vi "PassWrapper.vi"(11 "cPass":bool) -> (2 "Perform?":bool, 3 "Subsystem:\nGround (T)\nElevated (F)":bool)   [LabVIEW 2013]
doc: "Determines which pass method to use and whether to actually call the pass VI.\n\nAccepts the raw controller input (<B>cPass</B>).\nA <B>single</B> button press will select the <B>Ground Pass</B> (True).\nA <B>double</B> button press (i.e. double click) will select the <B>Elevated Pass</B> (False).\nAfter a small delay (250 ms), the VI will output True from <B>Perform?</B>, indicating input can be passed to the Toggle / Pass vi (in a nested case structure)."
uses:
  PassState.ctl
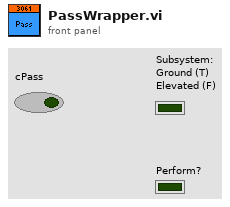
[diagram p1: front panel]
types:
  T1 = typedef "PassState.ctl" = enum16{"Idle", "SingleClick", "DoubleClick", "SelectPass", "Do"}
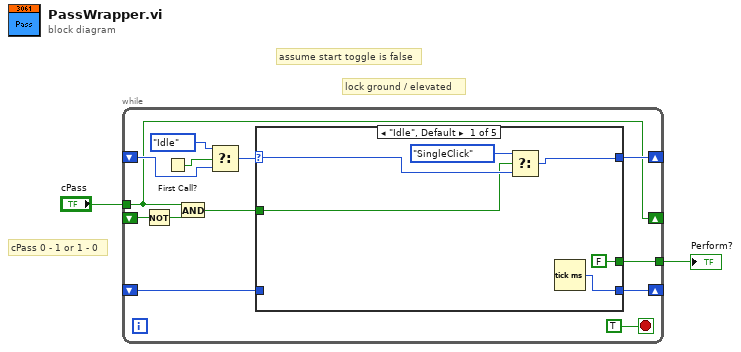
[diagram p0: block diagram]
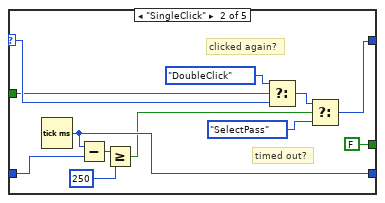
[diagram p2: hidden frame]
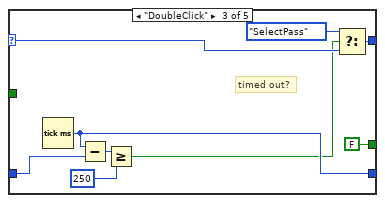
[diagram p3: hidden frame]
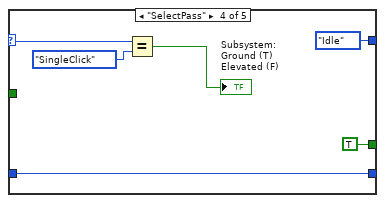
[diagram p4: hidden frame]
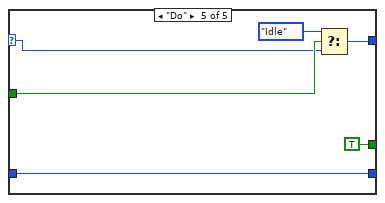
[diagram p5: hidden frame]
diagram:
  # "cPass 0 - 1 or 1 - 0"
  # "assume start toggle is false"
  # "lock ground / elevated"
  n1 = while {
    shift-right: [w10] -> _
    shift-left: _ -> [w11]
    shift-right: [w9] -> _
    shift-left: _ -> [w8]
    tunnel: [w7] -> w2
    shift-right: [w3] -> _
    shift-left: _ -> [w5]
    tunnel: "cPass" -> [w3]
    stop <- TRUE stop-if-true
    n2 = Not(x=w5) -> (.not. x?=w6:bool)
    n3 = First Call?() -> (First Call?: T/F=w14:bool)
    n4 = And(x=w3, y=w6) -> (x .and. y?=w4:bool)
    n5 = Select(t=PassState."Idle", s=w14, f=w11) -> (s? t:f=w12:T1)
    n6 = case shown="\"Idle\", Default" w12 {
      selector: w12 -> [w21 w23 w37 w46 w51]
      tunnel: [w20 w32 w38 PassState."Idle" w49] -> w10
      tunnel: [w18 w27 w39 w48 w53] -> w9
      tunnel: w8 -> [_ w28 w40 w48 w53]
      tunnel: [FALSE FALSE FALSE TRUE TRUE] -> w7
      tunnel: w4 -> [w16 w22 _ _ w52]
      frame "Idle", Default {
        n7 = Select(t=PassState."SingleClick", s=w16, f=w21) -> (s? t:f=w20:T1)
        n8 = Tick Count (ms)() -> (millisecond timer value=w18:u32)
      }
      frame "SingleClick" {
        # "timed out?"
        # "clicked again?"
        n9 = Tick Count (ms)() -> (millisecond timer value=w27:u32)
        n10 = Subtract(x=w27, y=w28) -> (x-y=w30:u32)
        n11 = Greater Or Equal?(x=w30, y=u32 250) -> (x >= y?=w26:bool)
        n12 = Select(t=PassState."DoubleClick", s=w22, f=w23) -> (s? t:f=w33:T1)
        n13 = Select(t=w33, s=w26, f=PassState."SelectPass") -> (s? t:f=w32:T1)
      }
      frame "DoubleClick" {
        # "timed out?"
        n14 = Tick Count (ms)() -> (millisecond timer value=w39:u32)
        n15 = Subtract(x=w39, y=w40) -> (x-y=w42:u32)
        n16 = Greater Or Equal?(x=w42, y=u32 250) -> (x >= y?=w35:bool)
        n17 = Select(t=PassState."SelectPass", s=w35, f=w37) -> (s? t:f=w38:T1)
      }
      frame "SelectPass" {
        n18 = Equal?(x=w46, y=PassState."SingleClick") -> (x = y?=→"Subsystem:\nGround (T)\nElevated (F)":bool)
      }
      frame "Do" {
        n19 = Select(t=PassState."Idle", s=w52, f=w51) -> (s? t:f=w49:T1)
      }
    }
  }
  "Perform?" <- w2
